vi "MT Open UART.vi"(11 "sCOM":string) -> (2 "function return":i32, 3 "sCOM out":string)   [LabVIEW 2014, in "MT_API.lvlib"]
doc: "MT_API INT32 __stdcall MT_Open_UART(char* sCOM);"
uses:
  MT_API.lvlib
  MT_API.dll
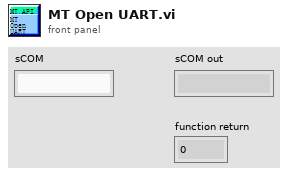
[diagram p1: front panel]
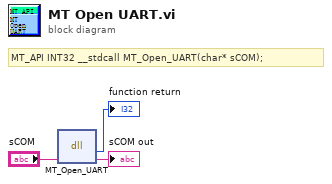
[diagram p0: block diagram]
diagram:
  # "MT_API INT32 __stdcall MT_Open_UART(char* sCOM);"
  n1 = dll-call lib="E:/Projects/LabView/MT_API/MT_API.*" fn="MT_Open_UART"("sCOM"="sCOM") -> (→"function return":i32, "sCOM"=→"sCOM out":string)  [unwired: 3 in, 2 out]
